vi "XY Graph Normally Positivise Plot.vi"(8 "error in (no error)":errorcluster, 11 "Plot in":cluster{"t Array":dbl[], "Array":dbl[]}) -> (0 "error out":errorcluster, 3 "Plot out":cluster{"t Array":dbl[], "Array":dbl[]})   [LabVIEW 2021, in "XY Graph Add-Ons.lvlib"]
uses:
  XY Graph Add-Ons.lvlib
  <vilib>/gmath/statdist.llb/Normal Random.vi
  <vilib>/gmath/NI_Gmath.lvlib
panel:
  # "see the License on the block diagram (Ctrl+E or Window:Show Block Diagram)"
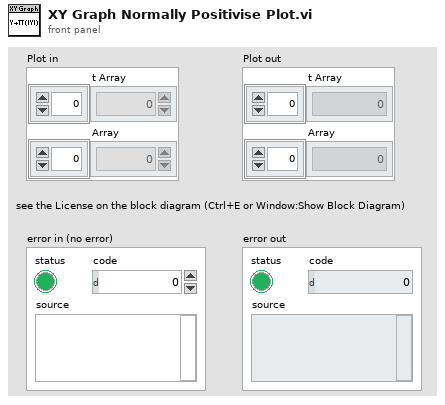
[diagram p1: front panel]
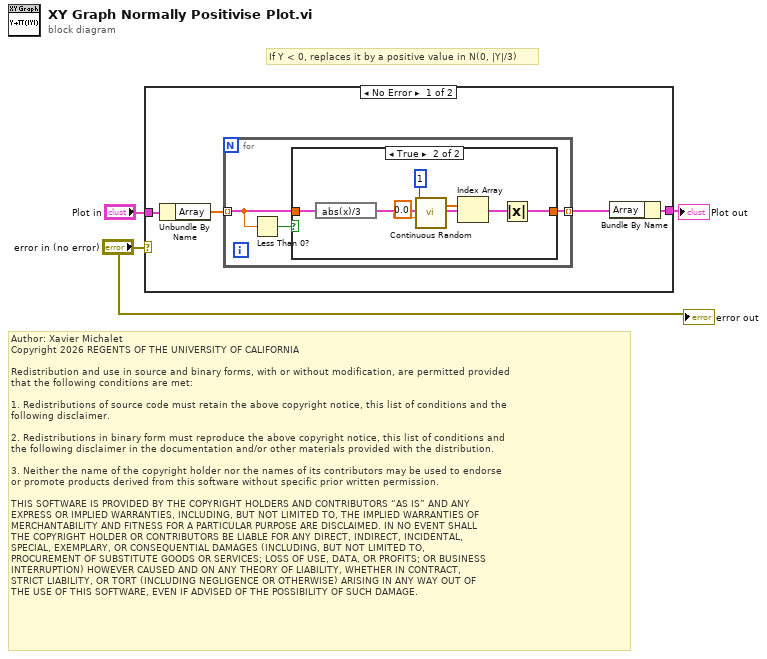
[diagram p0: block diagram]
diagram:
  # "Author: Xavier Michalet\nCopyright 2026 REGENTS OF THE UNIVERSITY OF CALIFORNIA\n\nRedistribution and use in source and binary forms, with or without modification, are permitted provided\nthat the following conditions are met:\n\n1. Redistributions of source code must retain the above copyright notice, this list of conditions and the\nfollowing disclaimer.\n\n2. Redistributions in binary form must reproduce the above copyright notice, this list of conditions and\nthe following disclaimer in the documentation and/or other materials provided with the distribution.\n\n3. Neither the name of the copyright holder nor the names of its contributors may be used to endorse \nor promote products derived from this software without specific prior written permission.\n\nTHIS SOFTWARE IS PROVIDED BY THE COPYRIGHT HOLDERS AND CONTRIBUTORS “AS IS” AND ANY \nEXPRESS OR IMPLIED WARRANTIES, INCLUDING, BUT NOT LIMITED TO, THE IMPLIED WARRANTIES OF\nMERCHANTABILITY AND FITNESS FOR A PARTICULAR PURPOSE ARE DISCLAIMED. IN NO EVENT SHALL\nTHE COPYRIGHT HOLDER OR CONTRIBUTORS BE LIABLE FOR ANY DIRECT, INDIRECT, INCIDENTAL, \nSPECIAL, EXEMPLARY, OR CONSEQUENTIAL DAMAGES (INCLUDING, BUT NOT LIMITED TO, \nPROCUREMENT OF SUBSTITUTE GOODS OR SERVICES; LOSS OF USE, DATA, OR PROFITS; OR BUSINESS\nINTERRUPTION) HOWEVER CAUSED AND ON ANY THEORY OF LIABILITY, WHETHER IN CONTRACT, \nSTRICT LIABILITY, OR TORT (INCLUDING NEGLIGENCE OR OTHERWISE) ARISING IN ANY WAY OUT OF\nTHE USE OF THIS SOFTWARE, EVEN IF ADVISED OF THE POSSIBILITY OF SUCH DAMAGE."
  # "If Y < 0, replaces it by a positive value in N(0, |Y|/3)"
  n1 = case shown="No Error" "error in (no error)" {
    tunnel: "Plot in" -> [w6 w19]
    tunnel: [w4 w19] -> w2
    frame No Error {
      n2 = Unbundle By Name(w6) -> ("Array"=w7:dbl[])
      n3 = for {
        tunnel: w7 -> [w9] mode=indexing
        tunnel: [w8] -> w5 mode=indexing
        n4 = Less Than 0?(x=w9) -> (x < 0?=w10:bool)
        n5 = case shown="True" w10 {
          tunnel: w9 -> [w11 w18]
          tunnel: [w11 w12] -> w8
          frame False {
          }
          frame True {
            n6 = expression code="abs(x)/3"(w18) -> (w17:dbl)
            n7 = call-poly <vilib>:"Continuous Random.vi"("std"=w17, "mean"=0.0, "samples"=1) -> ("normal random data"=w14:dbl[])  [unwired: 7 in, 1 out]
            n8 = Index Array(array=w14) -> (element=w13:dbl)  [unwired: 1 in]
            n9 = Absolute Value(x=w13) -> (abs(x)=w12:dbl)
          }
        }
      }
      n10 = Bundle By Name(cluster=w6, "Array"=w5) -> (w4:cluster{"t Array":dbl[], "Array":dbl[]})
    }
    frame Error {
    }
  }
  "Plot out" <- w2
  "error out" <- "error in (no error)"
